vi "GenereteAbsolutleUnique2DArray.vi"(8 "Colums":i32=6, 11 "Rows":i32=3) -> (0 "2D Double Array":i32[][](array[numeric]), 3 "2D String Array":string[][](array[string]))   [LabVIEW 2023]
uses:
  <vilib>/numeric/Random Number (Range) U64.vi
  <vilib>/numeric/sub_Random U32.vi
panel:
  out "Repeated attempt":i32
  out "?":i32
  out "?":i32
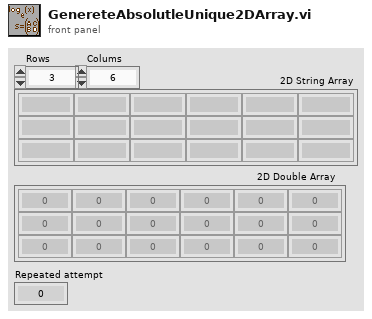
[diagram p1: front panel]
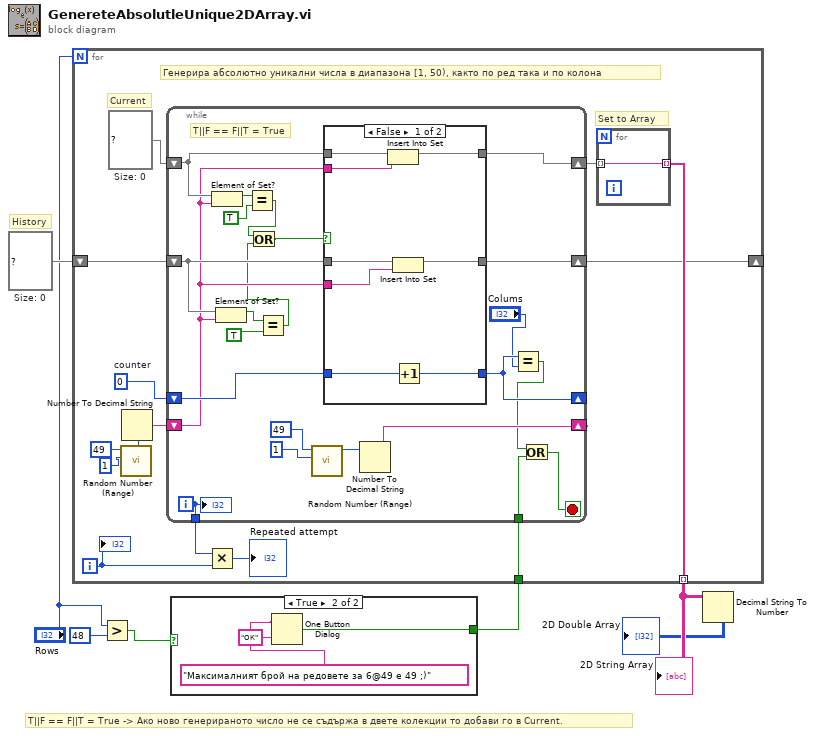
[diagram p0: block diagram]
diagram:
  w5 = set{string} {}  # Size: 0
  # "History"
  # "T||F == F||T = True -> Ако ново генерираното число не се съдържа в двете колекции то добави го в Current."
  n1 = Greater?(x="Rows", y=48) -> (0:w2:bool)
  n2 = case shown="True" w2 {
    selector: w2 -> [w8 _]
    tunnel: [w8 w9] -> w1
    frame False {
    }
    frame True {
      n3 = One Button Dialog(message="Максималният брой на редовете за 6@49 е 49 ;)", button name ("OK")="ОК") -> (true=w9:bool)
    }
  }
  n4 = for {
    N: "Rows" -> [_]
    tunnel: [w19] -> w7 mode=indexing
    shift-right: [w17] -> _
    shift-left: w5 -> [w16]
    tunnel: w1 -> [w12]
    i -> [w14]
    w18 = set{string} {}  # Size: 0
    w21 = 0  # counter
    # "Current"
    # "Генерира абсолютно уникални числа в диапазона [1, 50), както по ред така и по колона"
    # "Set to Array"
    n5 = call-poly <vilib>:"Random Number (Range).vi"("lower bound (0)"=u64 1, "upper bound (100)"=u64 49) -> ("number"=w25:u64)  [unwired: 9 in]
    n6 = Number To Decimal String(number=w25) -> (decimal integer string=w22:string)  [unwired: 1 in]
    n7 = while {
      shift-right: [w48] -> w20
      shift-left: w18 -> [w49]
      shift-right: [w41] -> _
      shift-left: w22 -> [w38]
      shift-right: [w46] -> _
      shift-left: w21 -> [w47]
      shift-right: [w40] -> w17
      shift-left: w16 -> [w39]
      tunnel: [w30] -> w15
      tunnel: w12 -> [w28]
      i -> [w30]
      stop <- w27 stop-if-true
      # "T||F == F||T = True"
      n8 = Element of Set?(10:w38, 11:w49) -> (3:w35:bool)
      n9 = Element of Set?(10:w38, 11:w39) -> (3:w37:bool)
      n10 = Equal?(x=w35, y=TRUE) -> (x = y?=w32:bool)
      n11 = Equal?(x=w37, y=TRUE) -> (x = y?=w33:bool)
      n12 = Or(x=w32, y=w33) -> (x .or. y?=w31:bool)
      n13 = call-poly <vilib>:"Random Number (Range).vi"("lower bound (0)"=u64 1, "upper bound (100)"=u64 49) -> ("number"=w44:u64)  [unwired: 9 in]
      n14 = case shown="False" w31 {
        tunnel: w49 -> [w57 w60]
        tunnel: w38 -> [w55 _]
        tunnel: [w56 w60] -> w48
        tunnel: w47 -> [w53 w59]
        tunnel: [w54 w59] -> w46
        tunnel: [w50 w58] -> w40
        tunnel: w38 -> [w52 _]
        tunnel: w39 -> [w51 w58]
        frame False {
          n15 = Insert Into Set(10:w55, 11:w57) -> (3:w56:set{string})  [unwired: 1 out]
          n16 = Insert Into Set(10:w52, 11:w51) -> (3:w50:set{string})  [unwired: 1 out]
          n17 = Increment(x=w53) -> (x+1=w54:i32)
        }
        frame True {
        }
      }
      n18 = Number To Decimal String(number=w44) -> (decimal integer string=w41:string)  [unwired: 1 in]
      n19 = Equal?(x=w46, y="Colums") -> (x = y?=w29:bool)
      n20 = Or(x=w29, y=w28) -> (x .or. y?=w27:bool)
      "?" <- w30
    }
    n21 = Multiply(x=w15, y=w14) -> (x*y=→"Repeated attempt":i32)
    n22 = for {
      tunnel: [w26] -> w19 mode=indexing
      tunnel: w20 -> [w26] mode=indexing
    }
    "?" <- w14
  }
  "2D String Array" <- w7
  n23 = Decimal String To Number(string=w7) -> (number=→"2D Double Array":i32[][])  [unwired: 2 in, 1 out]
